vi "Configure Current Limit.vi"(7 "Slave Address":i32=-1 min=-1 max=30 step=1, 8 "error":errorcluster, 9 "Settle (0 mS)":u32, 10 "Current Limit":dbl format="%.4f", 11 "VISA":refnum<visa-resource-name>) -> (0 "error out":errorcluster, 3 "VISA out":refnum<visa-resource-name>)   [LabVIEW 2019, in "TDK-Lambda GEN LAN Series.lvlib"]
doc: "Configure the current limit. The power supply output will go to this limit if the load causes Constant-Current operation.\n\nThis VI will wait for \"Settle\" milliseconds after setting the limit to allow the output to reach the new setting. If unwired, there is no delay"
uses:
  <instrlib>/TDK-Lambda GEN LAN Series/TDK-Lambda GEN LAN Series.lvlib
panel:
  # "TDK-Lambda Genesys \n   LAN\n  DC Power Supplies"
  # "Set the Current Limit"
  # "(c) 2019 TDK-Lambda.  ALL RIGHTS RESERVED."
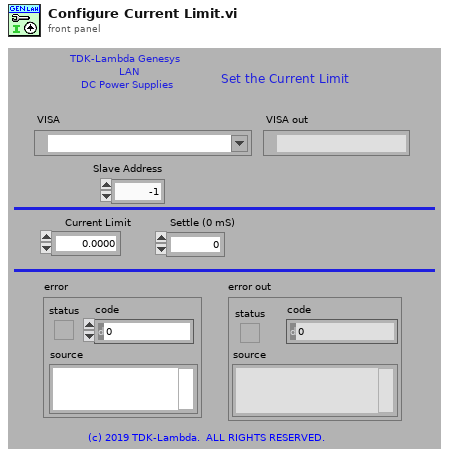
[diagram p1: front panel]
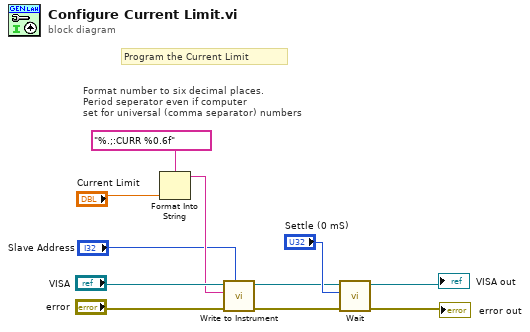
[diagram p0: block diagram]
diagram:
  # "Format number to six decimal places.\nPeriod seperator even if computer \nset for universal (comma separator) numbers"
  # "Program the Current Limit"
  n1 = Format Into String(format string="%.;:CURR %0.6f", "Current Limit") -> (resulting string=w4:string)  [unwired: 2 in, 1 out]
  n2 = call <instrlib>:"Write to Instrument.vi"("Slave Address"="Slave Address", "error"="error", "Command"=w4, "VISA"="VISA") -> ("error out"=w6:errorcluster, "VISA out"=w7:refnum<visa-resource-name>)  [unwired: 6 in]
  n3 = call <instrlib>:"Wait.vi"("error"=w6, "Delay (20 mS)"="Settle (0 mS)", "VISA"=w7) -> ("error out"=→"error out":errorcluster, "VISA out"=→"VISA out":refnum<visa-resource-name>)  [unwired: 7 in]
